vi "Configure Channel.vi"(7 "Chan Parameters":T1={"Channel"=1, "Chan State"=TRUE, "Chan Sync Source"=0, "Chan Gate Logic"=enum."Disabled", "Chan Mode"=enum."Normal", "Chan Wait #"=0, "Chan Delay"=2e-07, "Chan Width"=1e-06, "Chan Burst #"=10, "Chan DC On"=10, "Chan DC Off"=10, "Chan Polarity"=FALSE, "Chan MUX Value"=-1, "Chan Level Out"=enum."Adjustable", "Chan Lev Adjust"=9.0, "Chan Gate Mode"=enum."Disabled"} {"Chan Sync Source" items=["System (To)", "Channel A", "Channel B", "Channel C", "Channel D", "Channel E", "Channel F", "Channel G", "Channel H"]; "Chan Width" format="%.3p"; "Chan Delay" format="%.3p"; "Chan Lev Adjust" format="%.3p"; "Channel" items=["Channel A"=1, "Channel B"=2, "Channel C"=3, "Channel D"=4, "Channel E"=5, "Channel F"=6, "Channel G"=7, "Channel H"=8]}, 8 "error in (no error)":errorcluster, 11 "VISA resource name":refnum<visa-resource-name>="QCpulseGen") -> (0 "error out":errorcluster, 3 "VISA resource name out":refnum<visa-resource-name>)   [LabVIEW 2012]
doc: "This VI demonstrates how to use the \"All Chan Parameters.ctl\" and individual configuration functions to configure a channel.\n\nThe parameters \"Burst #\", \"Divide #\", and \"Adjustable\" are only updated when operating in the corresponding mode."
uses:
  Channel Parameters.ctl
  Public/Configure/Configure Chan Mode (Normal).vi
  Public/Configure/Configure Chan Mode (Single Shot).vi
  Public/Configure/Configure Chan Mode (Duty Cycle).vi
  Public/Configure/Configure Chan Mode (Burst).vi
  Quantum Composers 9000 Series.lvlib
panel:
  # "The parameters \"Burst #\", \"DC On\", \"DC Off\", and \"Adjustable\" are only updated when operating in the corresponding mode."
  # "Input"
  # "Normal\nSingle\nBurst"
  # "Burst"
  # "Duty Cycle"
  # "Output"
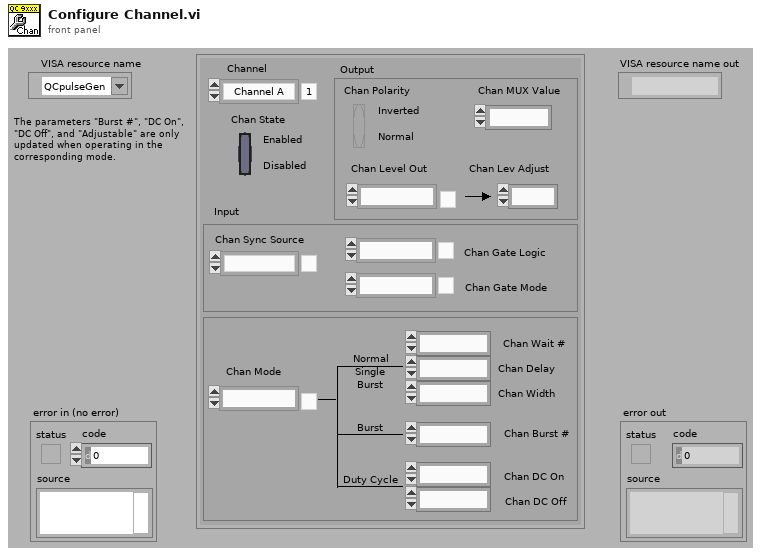
[diagram p1: front panel]
types:
  T1 = typedef "Channel Parameters.ctl" = cluster{"Channel":i32, "Chan State":bool, "Chan Sync Source":i32, "Chan Gate Logic":enum16{"Disabled", "Low", "High"}, "Chan Mode":enum16{"Normal", "Single", "Burst", "Duty Cycle"}, "Chan Wait #":i32, "Chan Delay":dbl, "Chan Width":dbl, "Chan Burst #":i32, "Chan DC On":i32, "Chan DC Off":i32, "Chan Polarity":bool, "Chan MUX Value":i32, "Chan Level Out":enum16{"TTL", "Adjustable", "35 Volt", "Optical"}, "Chan Lev Adjust":dbl, "Chan Gate Mode":enum16{"Disabled", "Pulse Inhibit", "Output Inhibit"}}
  T2 = enum16{"Disabled", "Pulse Inhibit", "Output Inhibit"}
  T3 = enum16{"Normal", "Single", "Burst", "Duty Cycle"}
  T4 = enum16{"TTL", "Adjustable", "35 Volt", "Optical"}
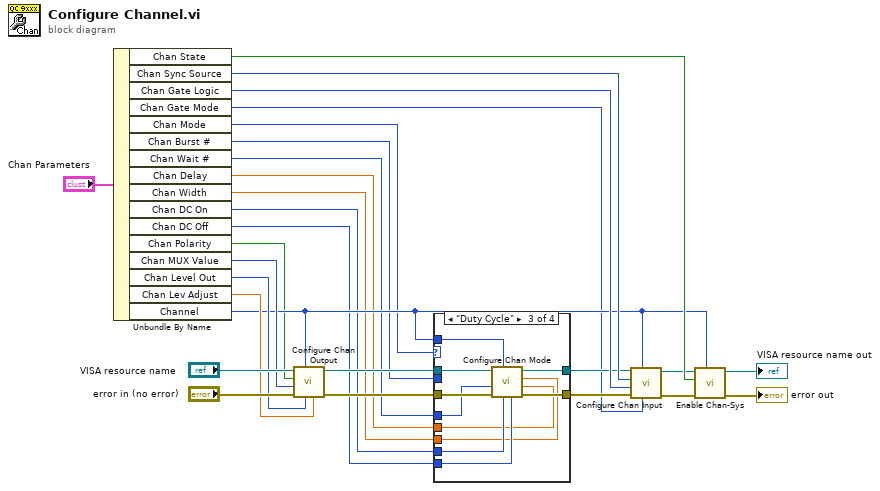
[diagram p0: block diagram]
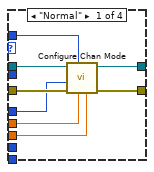
[diagram p2: hidden frame]
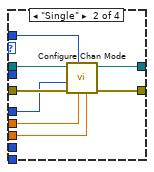
[diagram p3: hidden frame]
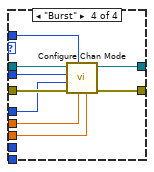
[diagram p4: hidden frame]
diagram:
  n1 = Unbundle By Name("Chan Parameters") -> ("Chan State"=w19:bool, "Chan Sync Source"=w18:i32, "Chan Gate Logic"=w17:enum16{"Disabled", "Low", "High"}, "Chan Gate Mode"=w1:T2, "Chan Mode"=w13:T3, "Chan Burst #"=w3:i32, "Chan Wait #"=w4:i32, "Chan Delay"=w7:dbl, "Chan Width"=w8:dbl, "Chan DC On"=w6:i32, "Chan DC Off"=w5:i32, "Chan Polarity"=w2:bool, "Chan MUX Value"=w22:i32, "Chan Level Out"=w21:T4, "Chan Lev Adjust"=w20:dbl, "Channel"=w14:i32)
  n2 = call "Configure Chan Output.vi"("Adjustable (5 Volts)"=w20, "Level (TTL)"=w21, "Channel (1:Chan A)"=w14, "error in (no error)"="error in (no error)", "MUX Value (-1)"=w22, "Polarity (F:Normal)"=w2, "VISA resource name"="VISA resource name") -> ("error out"=w11:errorcluster, "VISA resource name out"=w12:refnum<visa-resource-name>)  [unwired: 1 in, 2 out]
  n3 = case shown="\"Duty Cycle\"" w13 {
    tunnel: w14 -> [w35 w43 w53 w58]
    tunnel: w12 -> [w34 w42 w52 w62]
    tunnel: w11 -> [w33 w41 w51 w61]
    tunnel: [w32 w40 w50 w60] -> w10
    tunnel: [w31 w39 w49 w59] -> w9
    tunnel: w7 -> [w29 w36 w44 w56]
    tunnel: w4 -> [w30 w38 w48 w57]
    tunnel: w8 -> [w28 w37 w45 w55]
    tunnel: w6 -> [_ _ w47 _]
    tunnel: w5 -> [_ _ w46 _]
    tunnel: w3 -> [_ _ _ w54]
    frame "Normal" {
      n4 = call-poly "Configure Chan Mode.vi"("Width (10 msec)"=w28, "Delay (10 msec)"=w29, "Channel (1:Chan A)"=w35, "error in (no error)"=w33, "Wait # (0)"=w30, "VISA resource name"=w34) -> ("error out"=w31:errorcluster, "VISA resource name out"=w32:refnum<visa-resource-name>)  [unwired: 1 in, 3 out]
    }
    frame "Single" {
      n5 = call-poly "Configure Chan Mode.vi"("Width (10 msec)"=w37, "Delay (10 msec)"=w36, "Channel (1:Chan A)"=w43, "error in (no error)"=w41, "Wait # (0)"=w38, "VISA resource name"=w42) -> ("error out"=w39:errorcluster, "VISA resource name out"=w40:refnum<visa-resource-name>)  [unwired: 1 in, 3 out]
    }
    frame "Duty Cycle" {
      n6 = call-poly "Configure Chan Mode.vi"("Delay (10 msec)"=w44, "Width (10 msec)"=w45, "Chan DC Off (10)"=w46, "Chan DC On (10)"=w47, "Channel (1:Chan A)"=w53, "error in (no error)"=w51, "Wait # (0)"=w48, "VISA resource name"=w52) -> ("error out"=w49:errorcluster, "VISA resource name out"=w50:refnum<visa-resource-name>)  [unwired: 2 out]
    }
    frame "Burst" {
      n7 = call-poly "Configure Chan Mode.vi"("Width (10 msec)"=w55, "Delay (10 msec)"=w56, "Channel (1:Chan A)"=w58, "error in (no error)"=w61, "Wait # (0)"=w57, "Burst # (10)"=w54, "VISA resource name"=w62) -> ("error out"=w59:errorcluster, "VISA resource name out"=w60:refnum<visa-resource-name>)  [unwired: 3 out]
    }
  }
  n8 = call "Configure Chan Input.vi"("Gate Mode (0:Disabled)"=w1, "Channel (1:Chan A)"=w14, "error in (no error)"=w9, "Gate Logic (0:Disabled)"=w17, "Sync Source (0:To)"=w18, "VISA resource name"=w10) -> ("error out"=w15:errorcluster, "VISA resource name out"=w16:refnum<visa-resource-name>)  [unwired: 4 out]
  n9 = call "Enable Chan-Sys.vi"("Channel (1:Chan A)"=w14, "error in (no error)"=w15, "State (T:Enabled)"=w19, "VISA resource name"=w16) -> ("error out"=→"error out":errorcluster, "VISA resource name out"=→"VISA resource name out":refnum<visa-resource-name>)  [unwired: 6 out]
